vi "Gen - Front Panel Size.vi"(8 "Error In":errorcluster, 11 "This VI":refnum<vi>) -> (0 "Error Out":errorcluster)   [LabVIEW 2020]
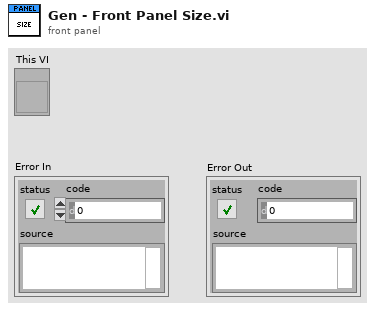
[diagram p1: front panel]
types:
  T1 = typedef "LVBoundsTypeDef.ctl" = cluster{"Width":u32, "Height":u32}
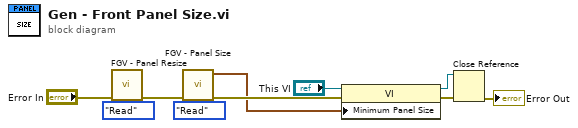
[diagram p0: block diagram]
diagram:
  n1 = call "FGV - Panel Resize.vi"("Action"=enum16{"Read", "Write"}."Read", "Error In"="Error In") -> ("Error Out"=w4:errorcluster)  [unwired: 8 in, 1 out]
  n2 = call "FGV - Panel Size.vi"("Action"=enum16{"Read", "Write"}."Read", "Error In"=w4) -> ("Error Out"=w10:errorcluster, "Size Out"=w8:T1)  [unwired: 8 in]
  n3 = property class="VI"(reference="This VI", error in=w10, "Minimum Panel Size"=w8) -> (reference out=w1:refnum<vi>, error out=w2:errorcluster)
  n4 = Close Reference(reference=w1, error in (no error)=w2) -> (error out=→"Error Out":errorcluster)
